vi "Feedback.vi"(8 "error in (no error)":errorcluster, 11 "UDP Reader in":refnum<class "UDP Reader.lvclass">) -> (0 "error out":errorcluster, 3 "UDP Reader out":refnum<class "UDP Reader.lvclass">)   [LabVIEW 2022 SP3, in "UDP Reader.lvlib" / "UDP Reader.lvclass"]
uses:
  UDP Reader.lvclass
  C:/Program Files (x86)/National Instruments/LabVIEW 2022/vi.lib/ActorFramework/Actor/Actor.lvclass
  <vilib>/ActorFramework/Actor/Actor.lvclass/Actor.ctl
  UDP Reader.lvclass/UDP Reader.ctl
  UDP Data Receiver/UDP Data Receiver Messages/RX Msg/RX Msg.lvclass/RX Msg.ctl
  <vilib>/ActorFramework/Message Enqueuer/Message Enqueuer.lvclass/Message Enqueuer.ctl
  <vilib>/ActorFramework/Message Enqueuer/Enqueue.vi
  UDP Data Receiver/UDP Data Receiver Messages/RX Msg/RX Msg.lvclass
  C:/Program Files (x86)/National Instruments/LabVIEW 2022/vi.lib/ActorFramework/Message/Message.lvclass
  <vilib>/ActorFramework/Message Priority Queue/Priority Enqueue.vi
  <vilib>/ActorFramework/Actor/Actor.lvclass
panel:
  out "RX":bool
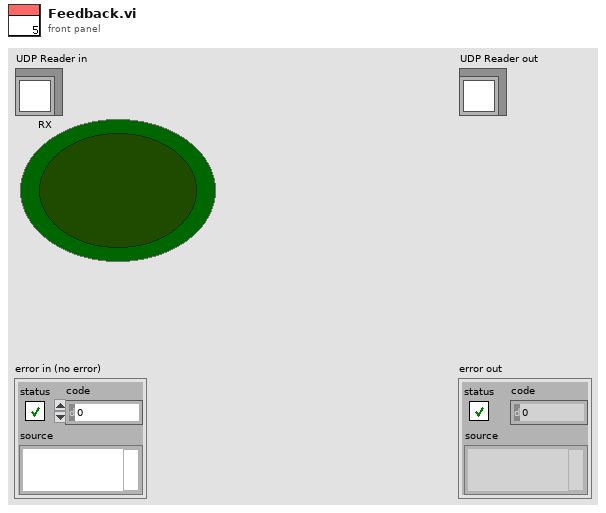
[diagram p1: front panel]
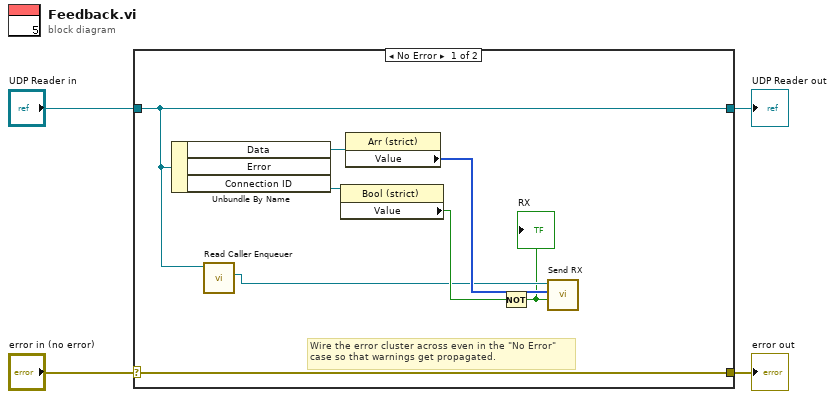
[diagram p0: block diagram]
diagram:
  n1 = case shown="No Error" "error in (no error)" {
    selector: "error in (no error)" -> [w12 w14]
    tunnel: [w12 w14] -> w3
    tunnel: [w9 w13] -> w1
    tunnel: "UDP Reader in" -> [w9 w13]
    frame No Error {
      # "Wire the error cluster across even in the \"No Error\"\ncase so that warnings get propagated."
      n2 = Unbundle By Name(w9) -> ("Data"=w10:refnum<vi>, "Error"=w11:refnum<vi>)  [unwired: 1 out]
      n3 = call <vilib>:"Read Caller Enqueuer.vi"("Actor"=w9) -> ("Caller Enqueuer"=w6:refnum<class "Message Enqueuer.lvclass">)  [unwired: 10 in]
      n4 = property class="Bool (strict)"(reference=w11) -> ("Value"=w7:bool)  [unwired: 1 in, 2 out]
      n5 = property class="Arr (strict)"(reference=w10) -> ("Value"=w8:u8[])  [unwired: 1 in, 2 out]
      n6 = Not(x=w7) -> (.not. x?=w5:bool)
      "RX" <- w5
      n7 = call "Send RX.vi"("RX"=w5, "Data"=w8, "Message Enqueuer"=w6) -> ()  [unwired: 7 in, 2 out]
    }
    frame Error {
    }
  }
  "error out" <- w3
  "UDP Reader out" <- w1
